vi "Get Wavelength.vi"(8 "error in (no error)":errorcluster, 11 "Simulated-Topas in":refnum<class "Simulated-Topas.lvclass">) -> (0 "error out":errorcluster, 2 "Wavelength":dbl, 3 "Simulated-Topas out":refnum<class "Simulated-Topas.lvclass">)   [LabVIEW 2019, in "Simulated-Topas.lvclass"]
uses:
  Simulated-Topas.lvclass
  Simulated-Topas.lvclass/Simulated-Topas.ctl
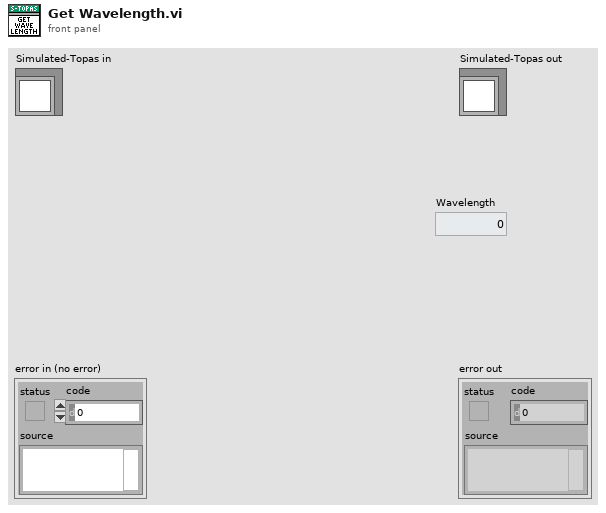
[diagram p1: front panel]
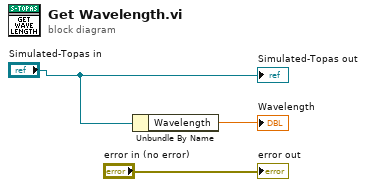
[diagram p0: block diagram]
diagram:
  n1 = Unbundle By Name("Simulated-Topas in") -> ("Wavelength"=→"Wavelength":dbl)
  "error out" <- "error in (no error)"
  "Simulated-Topas out" <- "Simulated-Topas in"
